vi "CorrectionThermistance.vi"(10 "Input Data":dbl[](array[numeric])) -> (2 "Data corrected":dbl[](array[numeric]))   [LabVIEW 2018]
uses:
  <vilib>/Analysis/NI_AALBase.lvlib
  <vilib>/Analysis/baseanly.llb/Mean (DBL).vi
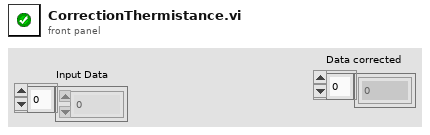
[diagram p1: front panel]
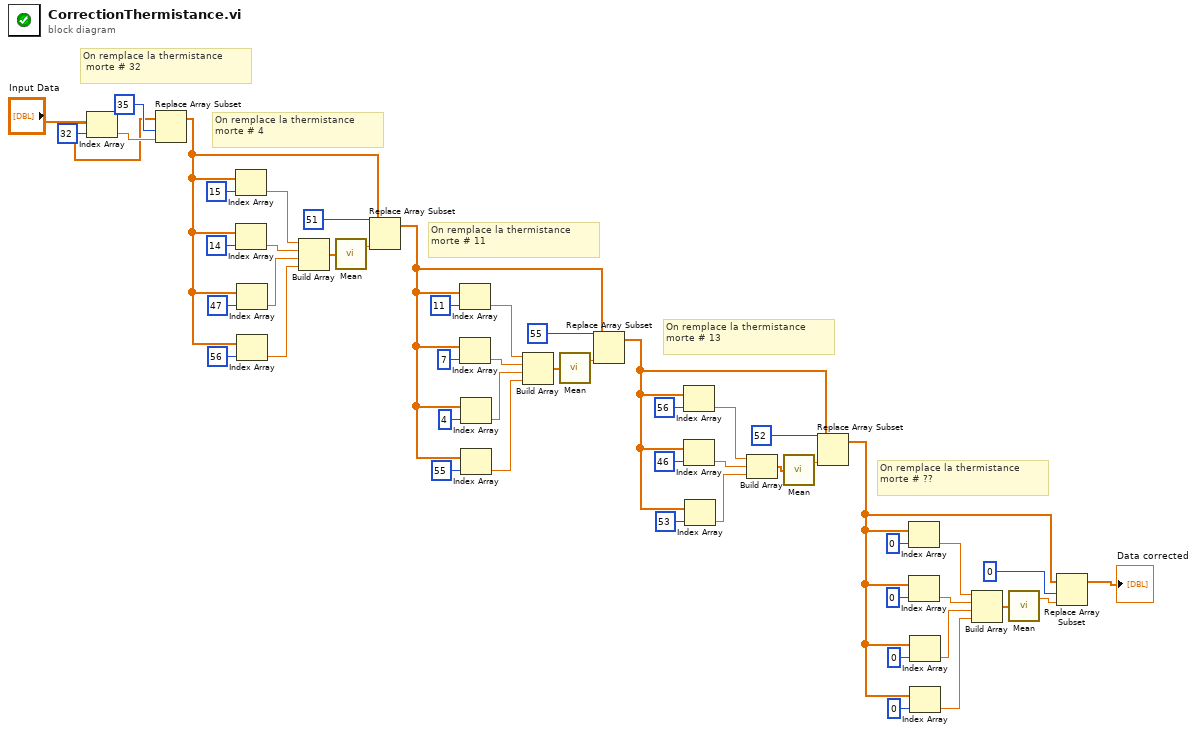
[diagram p0: block diagram]
diagram:
  # "On remplace la thermistance\nmorte # ??"
  # "On remplace la thermistance\nmorte # 13"
  # "On remplace la thermistance\nmorte # 11"
  # "On remplace la thermistance\nmorte # 4"
  # "On remplace la thermistance\n morte # 32"
  n1 = Index Array(array="Input Data", index=32) -> (element=w49:dbl)
  n2 = Replace Array Subset(array="Input Data", new element=w49, index=35) -> (w36:dbl[])
  n3 = Index Array(array=w36, index=15) -> (element=w43:dbl)
  n4 = Index Array(array=w36, index=14) -> (element=w42:dbl)
  n5 = Index Array(array=w36, index=47) -> (element=w41:dbl)
  n6 = Index Array(array=w36, index=56) -> (element=w40:dbl)
  n7 = Build Array(w43, w42, w41, w40) -> (w39:dbl[])
  n8 = call-poly <vilib>:"Mean.vi"("X"=w39) -> ("mean"=w38:dbl)  [unwired: 1 out]
  n9 = Replace Array Subset(array=w36, new element=w38, index=51) -> (w24:dbl[])
  n10 = Index Array(array=w24, index=11) -> (element=w31:dbl)
  n11 = Index Array(array=w24, index=7) -> (element=w30:dbl)
  n12 = Index Array(array=w24, index=4) -> (element=w29:dbl)
  n13 = Index Array(array=w24, index=55) -> (element=w28:dbl)
  n14 = Build Array(w31, w30, w29, w28) -> (w27:dbl[])
  n15 = call-poly <vilib>:"Mean.vi"("X"=w27) -> ("mean"=w26:dbl)  [unwired: 1 out]
  n16 = Replace Array Subset(array=w24, new element=w26, index=55) -> (w14:dbl[])
  n17 = Index Array(array=w14, index=56) -> (element=w20:dbl)
  n18 = Index Array(array=w14, index=46) -> (element=w19:dbl)
  n19 = Index Array(array=w14, index=53) -> (element=w18:dbl)
  n20 = Build Array(w20, w19, w18) -> (w17:dbl[])
  n21 = call-poly <vilib>:"Mean.vi"("X"=w17) -> ("mean"=w16:dbl)  [unwired: 1 out]
  n22 = Replace Array Subset(array=w14, new element=w16, index=52) -> (w1:dbl[])
  n23 = Index Array(array=w1, index=0) -> (element=w9:dbl)
  n24 = Index Array(array=w1, index=0) -> (element=w8:dbl)
  n25 = Index Array(array=w1, index=0) -> (element=w7:dbl)
  n26 = Index Array(array=w1, index=0) -> (element=w6:dbl)
  n27 = Build Array(w9, w8, w7, w6) -> (w5:dbl[])
  n28 = call-poly <vilib>:"Mean.vi"("X"=w5) -> ("mean"=w4:dbl)  [unwired: 1 out]
  n29 = Replace Array Subset(array=w1, new element=w4, index=0) -> (→"Data corrected":dbl[])
